vi "Swap.vi"(9 "Y":i32, 10 "X":i32, 11 "Unswapped Array":T1(array[cluster]) {"End" format="%<%.3X>T"; "Start" format="%<%.3X>T"}) -> (3 "Swapped Array":T1(array[cluster]) {"End" format="%<%.3X>T"; "Start" format="%<%.3X>T"})   [LabVIEW 2017]
panel:
  out "Min Index":u32
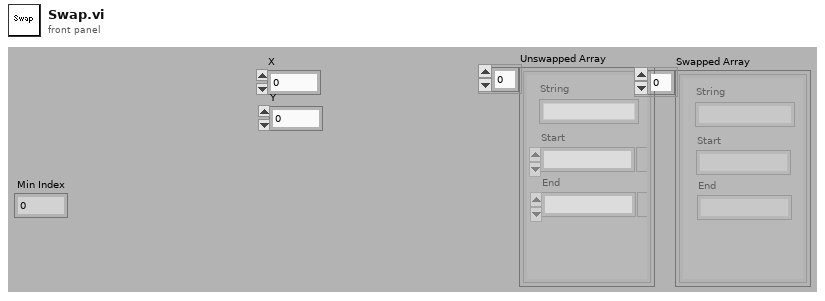
[diagram p1: front panel]
types:
  T1 = cluster{"String":string, "Start":timestamp, "End":timestamp}[]
  T2 = cluster{"String":string, "Start":timestamp, "End":timestamp}
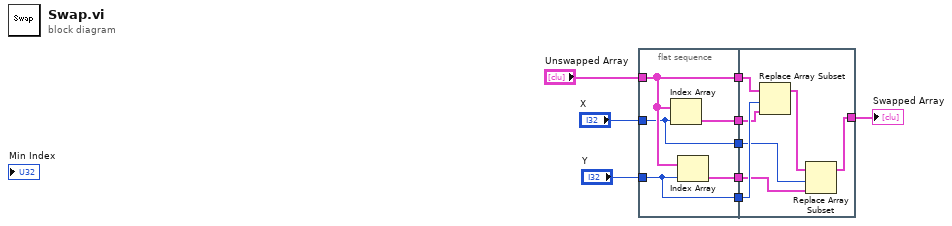
[diagram p0: block diagram]
diagram:
  n1 = flat-sequence {
    tunnel: "Unswapped Array" -> [w11]
    tunnel: [w11] -> w9
    tunnel: "Y" -> [w12]
    tunnel: "X" -> [w10]
    tunnel: [w14] -> w8
    tunnel: [w13] -> w7
    tunnel: [w10] -> w6
    tunnel: [w12] -> w5
    tunnel: w9 -> [w21]
    tunnel: w8 -> [w18]
    tunnel: w7 -> [w16]
    tunnel: w6 -> [w17]
    tunnel: w5 -> [w19]
    tunnel: [w15] -> w1
    frame #0 {
      n2 = Index Array(array=w11, index=w10) -> (element=w14:T2)
      n3 = Index Array(array=w11, index=w12) -> (element=w13:T2)
    }
    frame #1 {
      n4 = Replace Array Subset(array=w21, new element=w18, index=w19) -> (w20:T1)
      n5 = Replace Array Subset(array=w20, new element=w16, index=w17) -> (w15:T1)
    }
  }
  "Swapped Array" <- w1
